vi "EoTDetect.vi"(9 "Loops":i32=10, 10 "Tolerance":dbl=0.1, 11 "Sensor":dbl) -> (3 "EoT? (F)":bool)   [LabVIEW 2017]
uses:
  <vilib>/ptbypt/NI_PtbyPt.lvlib
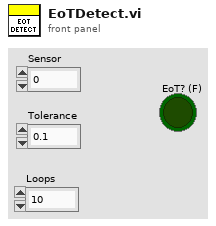
[diagram p1: front panel]
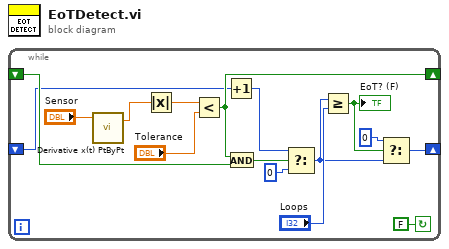
[diagram p0: block diagram]
diagram:
  n1 = while {
    shift-right: [w12] -> _
    shift-left: _ -> [w11]
    shift-right: [w2] -> _
    shift-left: _ -> [w8]
    stop <- FALSE continue-if-true
    n2 = call <vilib>:"Derivative x(t) PtByPt.vi"("x"="Sensor") -> ("dx/dt"=w14:dbl)  [unwired: 3 in, 1 out]
    n3 = Absolute Value(x=w14) -> (abs(x)=w15:dbl)
    n4 = Less?(x=w15, y="Tolerance") -> (x < y?=w12:bool)
    n5 = Increment(x=w8) -> (x+1=w7:i32)
    n6 = And(x=w12, y=w11) -> (x .and. y?=w10:bool)
    n7 = Select(t=w7, s=w10, f=0) -> (s? t:f=w1:i32)
    n8 = Greater Or Equal?(x=w1, y="Loops") -> (x >= y?=w4:bool)
    "EoT? (F)" <- w4
    n9 = Select(t=0, s=w4, f=w1) -> (s? t:f=w2:i32)
  }
